vi "update module id.vi"(8 "error in (no error)":errorcluster, 9 "New Id":string, 10 "Old Id":string, 11 "Standard Engine Configuration in":refnum<class "Standard Engine Configuration.lvclass">) -> (0 "error out":errorcluster, 3 "engine configuration out":refnum<class "engine configuration.lvclass">)   [LabVIEW 2013, in "Standard Engine Configuration.lvclass"]
uses:
  Standard Engine Configuration.lvclass
  <vilib>/NI/Module Execution Interface/Engine Configuration/engine configuration.lvclass
  Standard Engine Configuration.lvclass/Standard Engine Configuration.ctl
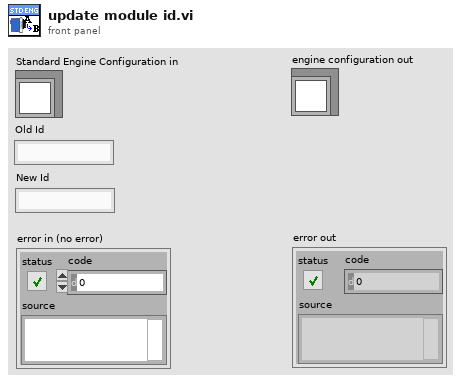
[diagram p1: front panel]
types:
  T1 = typedef "Standard Engine Configuration.lvclass/Module Specific Configuration.ctl" = cluster{"Module ID":string, "Module Decimation":T2, "error tag":string, "error responses":T3}
  T2 = typedef "Standard Engine Configuration.lvclass/Module Decimation.ctl" = cluster{"Decimation":u16, "Offset":u16, "sort order":i32, "async?":bool}
  T3 = typedef "Standard Engine Configuration.lvclass/error responses.ctl" = cluster{"unknown":T4, "trivial":T4, "critical":T4, "recoverable":T4}
  T4 = typedef "Standard Engine Configuration.lvclass/error options.ctl" = cluster{"clear":bool, "notify":bool, "log":bool, "remove module":bool, "abort engine":bool, "go to safe state":bool, "recover module":bool}
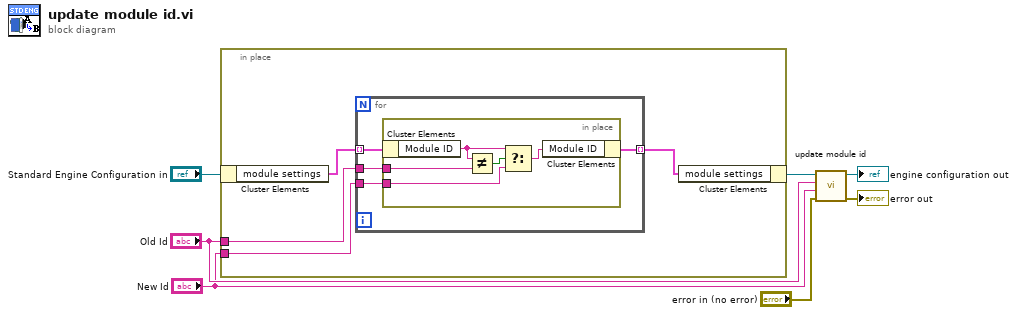
[diagram p0: block diagram]
diagram:
  n1 = in-place {
    in-place-border: "Old Id" -> [w9]
    in-place-border: "New Id" -> [w8]
    n2 = in-place-cluster #1("Standard Engine Configuration in") -> ("module settings"=w11:T1[])
    n3 = for {
      tunnel: w11 -> [w15] mode=indexing
      tunnel: [w14] -> w10 mode=indexing
      tunnel: w9 -> [w13]
      tunnel: w8 -> [w12]
      n4 = in-place {
        in-place-border: w13 -> [w18]
        in-place-border: w12 -> [w17]
        n5 = in-place-cluster #2(w15) -> ("Module ID"=w19:string)
        n6 = Not Equal?(x=w19, y=w18) -> (x != y?=w20:bool)
        n7 = Select(t=w19, s=w20, f=w17) -> (s? t:f=w16:string)
        n8 = in-place-cluster #2("Module ID"=w16) -> (w14:T1)
      }
    }
    n9 = in-place-cluster #1("module settings"=w10) -> (w3:refnum<class "Standard Engine Configuration.lvclass">)
  }
  n10 = call-parent "update module id.vi"("error in (no error)"="error in (no error)", "New Id"="New Id", "Old Id"="Old Id", "engine configuration in"=w3) -> ("error out"=→"error out":errorcluster, "engine configuration out"=→"engine configuration out":refnum<class "engine configuration.lvclass">)  [unwired: 6 in]
